vi "pointDensity.vi"(8 "Density":dbl=20.0, 9 "Pen in":bool[](array[boolean]), 10 "Y in":dbl[](array[numeric])=[10.0, 0.0, 5.0], 11 "X in":dbl[](array[numeric])=[0.0, 0.0, 10.0]) -> (1 "Pen out":bool[](array[boolean]), 2 "Y out":dbl[](array[numeric])=[9.5, 9.0, 8.5, 8.0, 7.5, 7.0, 6.5, 6.0, 5.5, 5.0, 4.5, 4.0, 3.5, 3.0, 2.5, 2.0, 1.5, 1.0, 0.5, 0.0, 0.22727272727272727, 0.45454545454545453, 0.6818181818181818, 0.9090909090909091, 1.1363636363636362, 1.3636363636363635, 1.5909090909090908, 1.8181818181818181, 2.0454545454545454, 2.2727272727272725, 2.4999999999999996, 2.7272727272727266, 2.9545454545454537, 3.1818181818181808, 3.409090909090908, 3.636363636363635, 3.863636363636362, 4.090909090909089, 4.318181818181817, 4.545454545454544, 4.772727272727272, 4.999999999999999], 3 "X out":dbl[](array[numeric])=[0.0, 0.0, 0.0, 0.0, 0.0, 0.0, 0.0, 0.0, 0.0, 0.0, 0.0, 0.0, 0.0, 0.0, 0.0, 0.0, 0.0, 0.0, 0.0, 0.0, 0.45454545454545453, 0.9090909090909091, 1.3636363636363635, 1.8181818181818181, 2.2727272727272725, 2.727272727272727, 3.1818181818181817, 3.6363636363636362, 4.090909090909091, 4.545454545454545, 4.999999999999999, 5.454545454545453, 5.909090909090907, 6.3636363636363615, 6.818181818181816, 7.27272727272727, 7.727272727272724, 8.181818181818178, 8.636363636363633, 9.090909090909088, 9.545454545454543, 9.999999999999998])   [LabVIEW 2014]
doc: "André Romero - 2016\nandretec@ifsc.usp.br\n\nIncrease density points of the vector"
panel:
  out "nearest integer value":ext=22.0
  out "size(s)":i32=42
  out "XY Graph Out":cluster{dbl[], dbl[]}(graph)={[0.0, 0.0, 0.0, 0.0, 0.0, 0.0, 0.0, 0.0, 0.0, 0.0, 0.0, 0.0, 0.0, 0.0, 0.0, 0.0, 0.0, 0.0, 0.0, 0.0, 0.45454545454545453, 0.9090909090909091, 1.3636363636363635, 1.8181818181818181, 2.2727272727272725, 2.727272727272727, 3.1818181818181817, 3.6363636363636362, 4.090909090909091, 4.545454545454545, 4.999999999999999, 5.454545454545453, 5.909090909090907, 6.3636363636363615, 6.818181818181816, 7.27272727272727, 7.727272727272724, 8.181818181818178, 8.636363636363633, 9.090909090909088, 9.545454545454543, 9.999999999999998], [9.5, 9.0, 8.5, 8.0, 7.5, 7.0, 6.5, 6.0, 5.5, 5.0, 4.5, 4.0, 3.5, 3.0, 2.5, 2.0, 1.5, 1.0, 0.5, 0.0, 0.22727272727272727, 0.45454545454545453, 0.6818181818181818, 0.9090909090909091, 1.1363636363636362, 1.3636363636363635, 1.5909090909090908, 1.8181818181818181, 2.0454545454545454, 2.2727272727272725, 2.4999999999999996, 2.7272727272727266, 2.9545454545454537, 3.1818181818181808, 3.409090909090908, 3.636363636363635, 3.863636363636362, 4.090909090909089, 4.318181818181817, 4.545454545454544, 4.772727272727272, 4.999999999999999]}
  out "XY Graph In":cluster{"X in":dbl[], "Y in":dbl[]}(graph)={"X in"=[0.0, 0.0, 10.0], "Y in"=[10.0, 0.0, 5.0]}
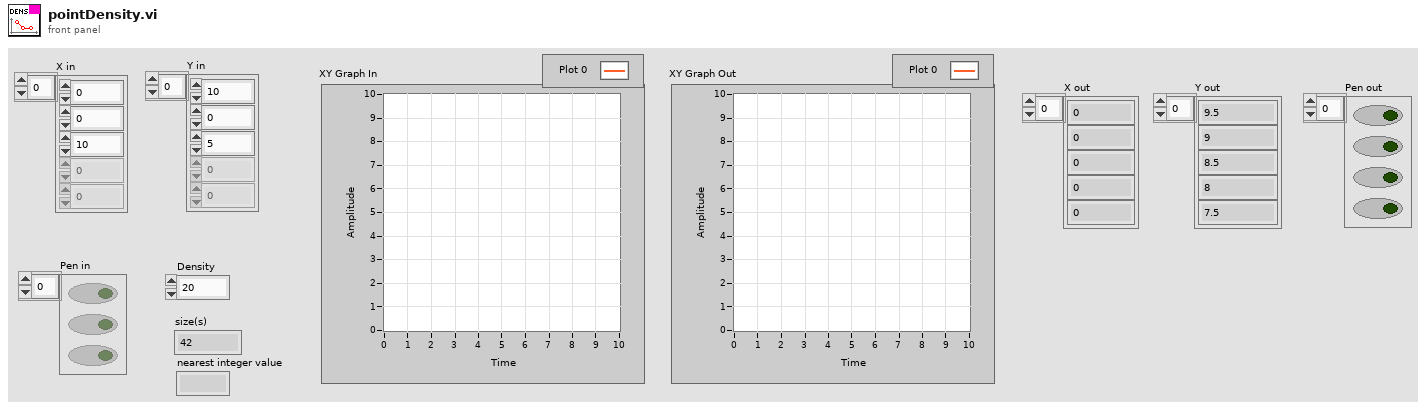
[diagram p1: front panel]
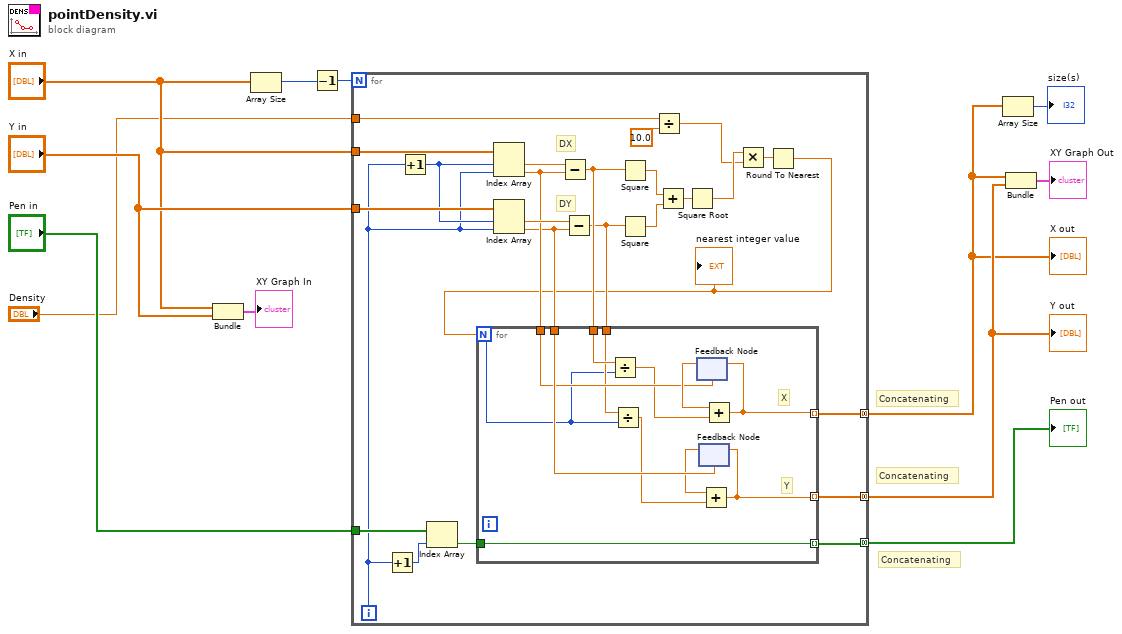
[diagram p0: block diagram]
diagram:
  # "Concatenating"
  # "Concatenating"
  # "Concatenating"
  n1 = Bundle("X in"="X in", "Y in"="Y in") -> (→"XY Graph In":cluster{"X in":dbl[], "Y in":dbl[]})  [unwired: 1 in]
  n2 = Array Size(array="X in") -> (size(s)=w11:i32)
  n3 = Decrement(x=w11) -> (x-1=w9:i32)
  n4 = for {
    N: w9 -> [_]
    tunnel: "X in" -> [w37]
    tunnel: "Y in" -> [w36]
    tunnel: "Pen in" -> [w28]
    tunnel: "Density" -> [w19]
    tunnel: [w17] -> w2 mode=concatenating
    tunnel: [w16] -> w4 mode=concatenating
    tunnel: [w15] -> w5 mode=concatenating
    i -> [w22]
    # "DY"
    # "DX"
    n5 = Increment(x=w22) -> (x+1=w27:i32)
    n6 = Increment(x=w22) -> (x+1=w23:i32)
    n7 = Index Array(array=w28, index=w27) -> (element=w29:bool)
    n8 = Index Array(array=w37, index #1=w23, index #2=w22) -> (element #1=w31:dbl, element #2=w21:dbl)
    n9 = Index Array(array=w36, index #1=w23, index #2=w22) -> (element #1=w30:dbl, element #2=w20:dbl)
    n10 = Subtract(x=w31, y=w21) -> (x-y=w26:dbl)
    n11 = Subtract(x=w30, y=w20) -> (x-y=w25:dbl)
    n12 = Square(x=w26) -> (x^2=w35:dbl)
    n13 = Square(x=w25) -> (x^2=w34:dbl)
    n14 = Divide(x=w19, y=10.0) -> (x/y=w14:dbl)
    n15 = Add(x=w35, y=w34) -> (x+y=w33:dbl)
    n16 = Square Root(x=w33) -> (sqrt(x)=w24:dbl)
    n17 = Multiply(x=w24, y=w14) -> (x*y=w32:dbl)
    n18 = Round To Nearest(number=w32) -> (nearest integer value=w18:dbl)
    "nearest integer value" <- w18
    n19 = for {
      N: w18 -> [w40]
      tunnel: w21 -> [w45]
      tunnel: w20 -> [w48]
      tunnel: w26 -> [w42]
      tunnel: w25 -> [w41]
      tunnel: w29 -> [w49]
      tunnel: [w49] -> w15 mode=indexing
      tunnel: [w39] -> w17 mode=indexing
      tunnel: [w38] -> w16 mode=indexing
      # "Y"
      # "X"
      n20 = Divide(x=w42, y=w40) -> (x/y=w44:dbl)
      n21 = Divide(x=w41, y=w40) -> (x/y=w43:dbl)
      n22 = feedback #1(w45) -> (w47:dbl)
      n23 = feedback #2(w48) -> (w46:dbl)
      n24 = Add(x=w46, y=w43) -> (x+y=w38:dbl)
      n25 = feedback-in #2(w38) -> ()
      n26 = Add(x=w47, y=w44) -> (x+y=w39:dbl)
      n27 = feedback-in #1(w39) -> ()
    }
  }
  "X out" <- w2
  "Y out" <- w4
  "Pen out" <- w5
  n28 = Array Size(array=w2) -> (size(s)=→"size(s)":i32)
  n29 = Bundle(w2, w4) -> (→"XY Graph Out":cluster{dbl[], dbl[]})  [unwired: 1 in]
